vi "GlobalGetBeamDiagnostics.vi"() -> ()   [LabVIEW 2013]
panel:
  in  "Get Beam Diagnostic":bool
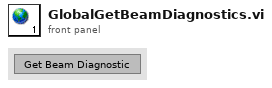
[diagram p1: front panel]
diagram:
